vi "DeferPanelUpdates.vi"(8 "error in (no error)":errorcluster, 10 "Defer Panel Updates?":bool, 11 "VI Ref":refnum<vi>) -> (0 "error out":errorcluster, 3 "VI Ref out":refnum<vi>)   [LabVIEW 2018]
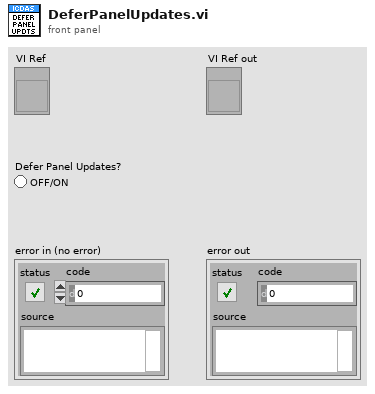
[diagram p1: front panel]
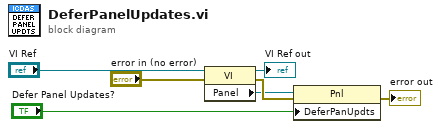
[diagram p0: block diagram]
diagram:
  n1 = property class="VI"(reference="VI Ref", error in="error in (no error)") -> (reference out=→"VI Ref out":refnum<vi>, error out=w5:errorcluster, "Panel"=w4:refnum<vi>)
  n2 = property class="Pnl"(reference=w4, error in=w5, "DeferPanUpdts"="Defer Panel Updates?") -> (error out=→"error out":errorcluster)  [unwired: 1 out]
